vi "CAN_parse_BMS_2_cell_voltages.vi"(11 "CAN message data":u8[](array[numeric])) -> ()   [LabVIEW 2018]
uses:
  Type_Def/TypeDef_BMSDatas.ctl
  Type_Def/TypeDef_BMSStatuss.ctl
  <vilib>/CANopenLib/CANOPEN.llb/CANopen Fetch from Data [U8].vi
  <vilib>/CANopenLib/CANOPEN.llb/CANopen Fetch from Data [U16].vi
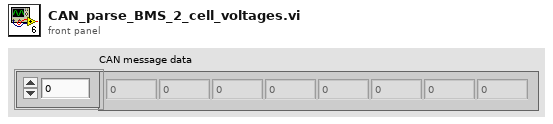
[diagram p1: front panel]
types:
  T1 = typedef "TypeDef_BMSDatas.ctl" = cluster{"Pack 1 Current (A)":dbl, "Pack 1 Voltage (V)":dbl, "Pack 1 Highest Temperature(C)":dbl, "BmsStatus1":T2, "Pack 2 Current (A)":dbl, "Pack 2 Voltage (V) ":dbl, "Pack 2 Highest Temperature(C) ":dbl, "BmsStatus 2":T2, "Pack 1 Cell Array (V)":dbl[], "Pack 2 Cell Array (V)":dbl[], "Pack 1 Lowest Temperature (C)":dbl, "Pack 1 Average Temperature (C)":dbl, "Pack 2 Average Temperature (C)":dbl, "Pack 2 Lowest Temperature (C)":dbl}
  T2 = typedef "TypeDef_BMSStatuss.ctl" = cluster{"isFault":bool, "isolationMonitoring":bool}
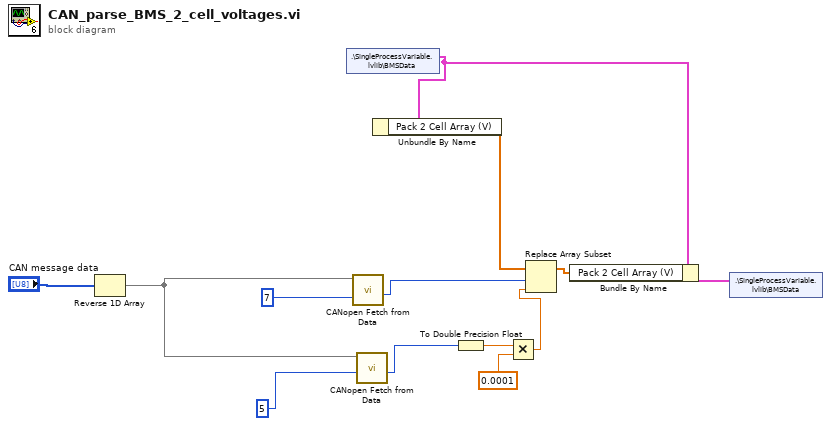
[diagram p0: block diagram]
diagram:
  n1 = Reverse 1D Array(array="CAN message data") -> (reversed array=w1:u8[])
  n2 = shared-variable ".\\SingleProcessVariable.lvlib\\BMSData"() -> (w4:T1)  [unwired: 1 in, 1 out]
  n3 = call-poly <vilib>:"CANopen Fetch from Data.vi"("offset (0)"=7, "CANopen data in"=w1) -> ("unsigned 8-bit integer"=w12:u8)  [unwired: 7 in, 2 out]
  n4 = call-poly <vilib>:"CANopen Fetch from Data.vi"("offset (0)"=5, "CANopen data in"=w1) -> ("unsigned 16-bit integer"=w9:u16)  [unwired: 7 in, 2 out]
  n5 = Unbundle By Name(w4) -> ("Pack 2 Cell Array (V)"=w11:dbl[])
  n6 = To Double Precision Float(number=w9) -> (double precision float=w7:dbl)
  n7 = Multiply(x=w7, y=0.0001) -> (x*y=w6:dbl)
  n8 = Replace Array Subset(array=w11, new element=w6, index=w12) -> (w5:dbl[])
  n9 = Bundle By Name(cluster=w4, "Pack 2 Cell Array (V)"=w5) -> (w3:T1)
  n10 = shared-variable ".\\SingleProcessVariable.lvlib\\BMSData"(w3) -> ()  [unwired: 1 in, 1 out]
